vi "PicoScope6000aExampleRapidBlockBulk.vi"() -> ()   [LabVIEW 2016]
uses:
  <vilib>/Waveform/DWDTOps.llb/DWDT Analog to Digital.vi
  PicoScope6000aLib/PicoScope6000aAnalogChannelSettings.ctl
  PicoScope6000aLib/PicoScope6000aDigitalChannelSettings.ctl
panel:
  in  "Digital Channels":T1={"Port 0 Settings "={"Enabled"=FALSE, "Hysteresis"=3, "Threshold Level (Volts)"=[1.0, 1.0, 1.0, 1.0, 1.0, 1.0, 1.0, 1.0]}, "Port 1 Settings"={"Enabled"=FALSE, "Hysteresis"=3, "Threshold Level (Volts)"=[1.0, 1.0, 1.0, 1.0, 1.0, 1.0, 1.0, 1.0]}} {"Port 1 Settings"."Threshold Level (Volts)" format="%#_4p"; "Port 1 Settings"."Hysteresis" items=["PICO_VERY_HIGH_400MV", "PICO_HIGH_200MV", "PICO_NORMAL_100MV", "PICO_LOW_50MV"]; "Port 0 Settings"."Threshold Level (Volts)" format="%#_4p"; "Port 0 Settings"."Hysteresis" items=["PICO_VERY_HIGH_400MV", "PICO_HIGH_200MV", "PICO_NORMAL_100MV", "PICO_LOW_50MV"]}
  in  "Channels":T2={"Channel A Settings "={"Enabled"=FALSE, "Coupling"=1, "Range"=0, "Analogue Offset"=0.0, "BandWidth"=0}, "Channel B Settings "={"Enabled"=FALSE, "Coupling"=1, "Range"=0, "Analogue Offset"=0.0, "BandWidth"=0}, "Channel C Settings "={"Enabled"=FALSE, "Coupling"=1, "Range"=0, "Analogue Offset"=0.0, "BandWidth"=0}, "Channel D Settings "={"Enabled"=FALSE, "Coupling"=1, "Range"=0, "Analogue Offset"=0.0, "BandWidth"=0}, "Channel E Settings "={"Enabled"=FALSE, "Coupling"=1, "Range"=0, "Analogue Offset"=0.0, "BandWidth"=0}, "Channel F Settings "={"Enabled"=FALSE, "Coupling"=1, "Range"=0, "Analogue Offset"=0.0, "BandWidth"=0}, "Channel G Settings "={"Enabled"=FALSE, "Coupling"=1, "Range"=0, "Analogue Offset"=0.0, "BandWidth"=0}, "Channel H Settings "={"Enabled"=FALSE, "Coupling"=1, "Range"=0, "Analogue Offset"=0.0, "BandWidth"=0}} {"Channel H Settings"."BandWidth" items=["Full"=0, "100kHz"=100000, "20kHz"=200000, "1MHz"=1000000, "20MHz"=20000000, "25MHz"=25000000, "50MHz"=50000000, "200MHz"=200000000, "250MHz"=250000000, "500MHz"=500000000]; "Channel H Settings"."Range" items=["10mV"=0, "20mV"=1, "50mV"=2, "100mV"=3, "200mV"=4, "500mV"=5, "1V"=6, "2V"=7, "5V"=8, "10V"=9, "20V"=10, "50V"=11, "100V"=12, "200V"=13, "x10_Probe_100mV"=32, "x10_Probe_200mV"=33, "x10_Probe_500mV"=34, "x10_Probe_1V"=35, "x10_Probe_2V"=36, "x10_Probe_5V"=37, "x10_Probe_10V"=38, "x10_Probe_20V"=39, "x10_Probe_50V"=40, "x10_Probe_100V"=41, "x10_Probe_200V"=42, "x10_Probe_500V"=43, "CURRENT_CLAMP_60A_2A"=10500, "CURRENT_CLAMP_60A_5A"=10501, "CURRENT_CLAMP_60A_10A"=10502, "CURRENT_CLAMP_60A_20A"=10503, "CURRENT_CLAMP_60A_50A"=10504, "CURRENT_CLAMP_60A_60A"=10505, "CURRENT_CLAMP_60A_V2_0_5A"=10600, "CURRENT_CLAMP_60A_V2_1A"=10601, "CURRENT_CLAMP_60A_V2_2A"=10602, "CURRENT_CLAMP_60A_V2_5A"=10603, "CURRENT_CLAMP_60A_V2_10A"=10604, "CURRENT_CLAMP_60A_V2_20A"=10605, "CURRENT_CLAMP_60A_V2_50A"=10606, "CURRENT_CLAMP_60A_V2_60A"=10607, "RESISTANCE_LEAD_NEG5_TO_20OHM"=7000, "RESISTANCE_LEAD_NEG50_TO_200OHM"=7001, "RESISTANCE_LEAD_NEG500_TO_2KOHM"=7002, "RESISTANCE_LEAD_NEG5K_TO_20KOHM"=7003, "RESISTANCE_LEAD_NEG50K_TO_LEAD_200KOHM"=7004, "RESISTANCE_LEAD_NEG500K_TO_LEAD_2MOHM"=7005, "RESISTANCE_LEAD_DIODE_TEST"=7006, "HT_NEG3_TO_5KV"=8950, "HT_NEG3_TO_10KV"=8951, "HT_NEG5_TO_20KV"=8952, "HT_NEG5_TO_50KV"=8953, "HT_NEG5_TO_100KV"=8954, "HT_NEG3_TO_5KV_INVERTED"=8955, "HT_NEG3_TO_10KV_INVERTED"=8956, "HT_NEG5_TO_20KV_INVERTED"=8957, "HT_NEG5_TO_50KV_INVERTED"=8958, "HT_NEG5_TO_100KV_INVERTED"=8959, "TEMPERATURE_NEG50_TO_150DEGC"=9000, "PRESSURE_SENSOR_-100k-150k_PASCALS"=9100, "PRESSURE_SENSOR_-100k_TO_400k_PASCALS"=9101, "PRESSURE_SENSOR_-200k_TO_800k_PASCALS"=9102, "PRESSURE_SENSOR_-400k_TO_1600k_PASCALS"=9103, "PRESSURE_SENSOR_-400k_TO_3400k_PASCALS"=9104, "PRESSURE_SENSOR_-150k_TO_1350k_PASCALS"=9105]; "Channel H Settings"."Coupling" items=["AC"=0, "DC 1M Ohm"=1, "DC 50 Ohm"=50]; "Channel G Settings"."BandWidth" items=["Full"=0, "100kHz"=100000, "20kHz"=200000, "1MHz"=1000000, "20MHz"=20000000, "25MHz"=25000000, "50MHz"=50000000, "200MHz"=200000000, "250MHz"=250000000, "500MHz"=500000000]; "Channel G Settings"."Range" items=["10mV"=0, "20mV"=1, "50mV"=2, "100mV"=3, "200mV"=4, "500mV"=5, "1V"=6, "2V"=7, "5V"=8, "10V"=9, "20V"=10, "50V"=11, "100V"=12, "200V"=13, "x10_Probe_100mV"=32, "x10_Probe_200mV"=33, "x10_Probe_500mV"=34, "x10_Probe_1V"=35, "x10_Probe_2V"=36, "x10_Probe_5V"=37, "x10_Probe_10V"=38, "x10_Probe_20V"=39, "x10_Probe_50V"=40, "x10_Probe_100V"=41, "x10_Probe_200V"=42, "x10_Probe_500V"=43, "CURRENT_CLAMP_60A_2A"=10500, "CURRENT_CLAMP_60A_5A"=10501, "CURRENT_CLAMP_60A_10A"=10502, "CURRENT_CLAMP_60A_20A"=10503, "CURRENT_CLAMP_60A_50A"=10504, "CURRENT_CLAMP_60A_60A"=10505, "CURRENT_CLAMP_60A_V2_0_5A"=10600, "CURRENT_CLAMP_60A_V2_1A"=10601, "CURRENT_CLAMP_60A_V2_2A"=10602, "CURRENT_CLAMP_60A_V2_5A"=10603, "CURRENT_CLAMP_60A_V2_10A"=10604, "CURRENT_CLAMP_60A_V2_20A"=10605, "CURRENT_CLAMP_60A_V2_50A"=10606, "CURRENT_CLAMP_60A_V2_60A"=10607, "RESISTANCE_LEAD_NEG5_TO_20OHM"=7000, "RESISTANCE_LEAD_NEG50_TO_200OHM"=7001, "RESISTANCE_LEAD_NEG500_TO_2KOHM"=7002, "RESISTANCE_LEAD_NEG5K_TO_20KOHM"=7003, "RESISTANCE_LEAD_NEG50K_TO_LEAD_200KOHM"=7004, "RESISTANCE_LEAD_NEG500K_TO_LEAD_2MOHM"=7005, "RESISTANCE_LEAD_DIODE_TEST"=7006, "HT_NEG3_TO_5KV"=8950, "HT_NEG3_TO_10KV"=8951, "HT_NEG5_TO_20KV"=8952, "HT_NEG5_TO_50KV"=8953, "HT_NEG5_TO_100KV"=8954, "HT_NEG3_TO_5KV_INVERTED"=8955, "HT_NEG3_TO_10KV_INVERTED"=8956, "HT_NEG5_TO_20KV_INVERTED"=8957, "HT_NEG5_TO_50KV_INVERTED"=8958, "HT_NEG5_TO_100KV_INVERTED"=8959, "TEMPERATURE_NEG50_TO_150DEGC"=9000, "PRESSURE_SENSOR_-100k-150k_PASCALS"=9100, "PRESSURE_SENSOR_-100k_TO_400k_PASCALS"=9101, "PRESSURE_SENSOR_-200k_TO_800k_PASCALS"=9102, "PRESSURE_SENSOR_-400k_TO_1600k_PASCALS"=9103, "PRESSURE_SENSOR_-400k_TO_3400k_PASCALS"=9104, "PRESSURE_SENSOR_-150k_TO_1350k_PASCALS"=9105]; "Channel G Settings"."Coupling" items=["AC"=0, "DC 1M Ohm"=1, "DC 50 Ohm"=50]; "Channel F Settings"."BandWidth" items=["Full"=0, "100kHz"=100000, "20kHz"=200000, "1MHz"=1000000, "20MHz"=20000000, "25MHz"=25000000, "50MHz"=50000000, "200MHz"=200000000, "250MHz"=250000000, "500MHz"=500000000]; "Channel F Settings"."Range" items=["10mV"=0, "20mV"=1, "50mV"=2, "100mV"=3, "200mV"=4, "500mV"=5, "1V"=6, "2V"=7, "5V"=8, "10V"=9, "20V"=10, "50V"=11, "100V"=12, "200V"=13, "x10_Probe_100mV"=32, "x10_Probe_200mV"=33, "x10_Probe_500mV"=34, "x10_Probe_1V"=35, "x10_Probe_2V"=36, "x10_Probe_5V"=37, "x10_Probe_10V"=38, "x10_Probe_20V"=39, "x10_Probe_50V"=40, "x10_Probe_100V"=41, "x10_Probe_200V"=42, "x10_Probe_500V"=43, "CURRENT_CLAMP_60A_2A"=10500, "CURRENT_CLAMP_60A_5A"=10501, "CURRENT_CLAMP_60A_10A"=10502, "CURRENT_CLAMP_60A_20A"=10503, "CURRENT_CLAMP_60A_50A"=10504, "CURRENT_CLAMP_60A_60A"=10505, "CURRENT_CLAMP_60A_V2_0_5A"=10600, "CURRENT_CLAMP_60A_V2_1A"=10601, "CURRENT_CLAMP_60A_V2_2A"=10602, "CURRENT_CLAMP_60A_V2_5A"=10603, "CURRENT_CLAMP_60A_V2_10A"=10604, "CURRENT_CLAMP_60A_V2_20A"=10605, "CURRENT_CLAMP_60A_V2_50A"=10606, "CURRENT_CLAMP_60A_V2_60A"=10607, "RESISTANCE_LEAD_NEG5_TO_20OHM"=7000, "RESISTANCE_LEAD_NEG50_TO_200OHM"=7001, "RESISTANCE_LEAD_NEG500_TO_2KOHM"=7002, "RESISTANCE_LEAD_NEG5K_TO_20KOHM"=7003, "RESISTANCE_LEAD_NEG50K_TO_LEAD_200KOHM"=7004, "RESISTANCE_LEAD_NEG500K_TO_LEAD_2MOHM"=7005, "RESISTANCE_LEAD_DIODE_TEST"=7006, "HT_NEG3_TO_5KV"=8950, "HT_NEG3_TO_10KV"=8951, "HT_NEG5_TO_20KV"=8952, "HT_NEG5_TO_50KV"=8953, "HT_NEG5_TO_100KV"=8954, "HT_NEG3_TO_5KV_INVERTED"=8955, "HT_NEG3_TO_10KV_INVERTED"=8956, "HT_NEG5_TO_20KV_INVERTED"=8957, "HT_NEG5_TO_50KV_INVERTED"=8958, "HT_NEG5_TO_100KV_INVERTED"=8959, "TEMPERATURE_NEG50_TO_150DEGC"=9000, "PRESSURE_SENSOR_-100k-150k_PASCALS"=9100, "PRESSURE_SENSOR_-100k_TO_400k_PASCALS"=9101, "PRESSURE_SENSOR_-200k_TO_800k_PASCALS"=9102, "PRESSURE_SENSOR_-400k_TO_1600k_PASCALS"=9103, "PRESSURE_SENSOR_-400k_TO_3400k_PASCALS"=9104, "PRESSURE_SENSOR_-150k_TO_1350k_PASCALS"=9105]; "Channel F Settings"."Coupling" items=["AC"=0, "DC 1M Ohm"=1, "DC 50 Ohm"=50]; "Channel E Settings"."BandWidth" items=["Full"=0, "100kHz"=100000, "20kHz"=200000, "1MHz"=1000000, "20MHz"=20000000, "25MHz"=25000000, "50MHz"=50000000, "200MHz"=200000000, "250MHz"=250000000, "500MHz"=500000000]; "Channel E Settings"."Range" items=["10mV"=0, "20mV"=1, "50mV"=2, "100mV"=3, "200mV"=4, "500mV"=5, "1V"=6, "2V"=7, "5V"=8, "10V"=9, "20V"=10, "50V"=11, "100V"=12, "200V"=13, "x10_Probe_100mV"=32, "x10_Probe_200mV"=33, "x10_Probe_500mV"=34, "x10_Probe_1V"=35, "x10_Probe_2V"=36, "x10_Probe_5V"=37, "x10_Probe_10V"=38, "x10_Probe_20V"=39, "x10_Probe_50V"=40, "x10_Probe_100V"=41, "x10_Probe_200V"=42, "x10_Probe_500V"=43, "CURRENT_CLAMP_60A_2A"=10500, "CURRENT_CLAMP_60A_5A"=10501, "CURRENT_CLAMP_60A_10A"=10502, "CURRENT_CLAMP_60A_20A"=10503, "CURRENT_CLAMP_60A_50A"=10504, "CURRENT_CLAMP_60A_60A"=10505, "CURRENT_CLAMP_60A_V2_0_5A"=10600, "CURRENT_CLAMP_60A_V2_1A"=10601, "CURRENT_CLAMP_60A_V2_2A"=10602, "CURRENT_CLAMP_60A_V2_5A"=10603, "CURRENT_CLAMP_60A_V2_10A"=10604, "CURRENT_CLAMP_60A_V2_20A"=10605, "CURRENT_CLAMP_60A_V2_50A"=10606, "CURRENT_CLAMP_60A_V2_60A"=10607, "RESISTANCE_LEAD_NEG5_TO_20OHM"=7000, "RESISTANCE_LEAD_NEG50_TO_200OHM"=7001, "RESISTANCE_LEAD_NEG500_TO_2KOHM"=7002, "RESISTANCE_LEAD_NEG5K_TO_20KOHM"=7003, "RESISTANCE_LEAD_NEG50K_TO_LEAD_200KOHM"=7004, "RESISTANCE_LEAD_NEG500K_TO_LEAD_2MOHM"=7005, "RESISTANCE_LEAD_DIODE_TEST"=7006, "HT_NEG3_TO_5KV"=8950, "HT_NEG3_TO_10KV"=8951, "HT_NEG5_TO_20KV"=8952, "HT_NEG5_TO_50KV"=8953, "HT_NEG5_TO_100KV"=8954, "HT_NEG3_TO_5KV_INVERTED"=8955, "HT_NEG3_TO_10KV_INVERTED"=8956, "HT_NEG5_TO_20KV_INVERTED"=8957, "HT_NEG5_TO_50KV_INVERTED"=8958, "HT_NEG5_TO_100KV_INVERTED"=8959, "TEMPERATURE_NEG50_TO_150DEGC"=9000, "PRESSURE_SENSOR_-100k-150k_PASCALS"=9100, "PRESSURE_SENSOR_-100k_TO_400k_PASCALS"=9101, "PRESSURE_SENSOR_-200k_TO_800k_PASCALS"=9102, "PRESSURE_SENSOR_-400k_TO_1600k_PASCALS"=9103, "PRESSURE_SENSOR_-400k_TO_3400k_PASCALS"=9104, "PRESSURE_SENSOR_-150k_TO_1350k_PASCALS"=9105]; "Channel E Settings"."Coupling" items=["AC"=0, "DC 1M Ohm"=1, "DC 50 Ohm"=50]; "Channel D Settings"."BandWidth" items=["Full"=0, "100kHz"=100000, "20kHz"=200000, "1MHz"=1000000, "20MHz"=20000000, "25MHz"=25000000, "50MHz"=50000000, "200MHz"=200000000, "250MHz"=250000000, "500MHz"=500000000]; "Channel D Settings"."Range" items=["10mV"=0, "20mV"=1, "50mV"=2, "100mV"=3, "200mV"=4, "500mV"=5, "1V"=6, "2V"=7, "5V"=8, "10V"=9, "20V"=10, "50V"=11, "100V"=12, "200V"=13, "x10_Probe_100mV"=32, "x10_Probe_200mV"=33, "x10_Probe_500mV"=34, "x10_Probe_1V"=35, "x10_Probe_2V"=36, "x10_Probe_5V"=37, "x10_Probe_10V"=38, "x10_Probe_20V"=39, "x10_Probe_50V"=40, "x10_Probe_100V"=41, "x10_Probe_200V"=42, "x10_Probe_500V"=43, "CURRENT_CLAMP_60A_2A"=10500, "CURRENT_CLAMP_60A_5A"=10501, "CURRENT_CLAMP_60A_10A"=10502, "CURRENT_CLAMP_60A_20A"=10503, "CURRENT_CLAMP_60A_50A"=10504, "CURRENT_CLAMP_60A_60A"=10505, "CURRENT_CLAMP_60A_V2_0_5A"=10600, "CURRENT_CLAMP_60A_V2_1A"=10601, "CURRENT_CLAMP_60A_V2_2A"=10602, "CURRENT_CLAMP_60A_V2_5A"=10603, "CURRENT_CLAMP_60A_V2_10A"=10604, "CURRENT_CLAMP_60A_V2_20A"=10605, "CURRENT_CLAMP_60A_V2_50A"=10606, "CURRENT_CLAMP_60A_V2_60A"=10607, "RESISTANCE_LEAD_NEG5_TO_20OHM"=7000, "RESISTANCE_LEAD_NEG50_TO_200OHM"=7001, "RESISTANCE_LEAD_NEG500_TO_2KOHM"=7002, "RESISTANCE_LEAD_NEG5K_TO_20KOHM"=7003, "RESISTANCE_LEAD_NEG50K_TO_LEAD_200KOHM"=7004, "RESISTANCE_LEAD_NEG500K_TO_LEAD_2MOHM"=7005, "RESISTANCE_LEAD_DIODE_TEST"=7006, "HT_NEG3_TO_5KV"=8950, "HT_NEG3_TO_10KV"=8951, "HT_NEG5_TO_20KV"=8952, "HT_NEG5_TO_50KV"=8953, "HT_NEG5_TO_100KV"=8954, "HT_NEG3_TO_5KV_INVERTED"=8955, "HT_NEG3_TO_10KV_INVERTED"=8956, "HT_NEG5_TO_20KV_INVERTED"=8957, "HT_NEG5_TO_50KV_INVERTED"=8958, "HT_NEG5_TO_100KV_INVERTED"=8959, "TEMPERATURE_NEG50_TO_150DEGC"=9000, "PRESSURE_SENSOR_-100k-150k_PASCALS"=9100, "PRESSURE_SENSOR_-100k_TO_400k_PASCALS"=9101, "PRESSURE_SENSOR_-200k_TO_800k_PASCALS"=9102, "PRESSURE_SENSOR_-400k_TO_1600k_PASCALS"=9103, "PRESSURE_SENSOR_-400k_TO_3400k_PASCALS"=9104, "PRESSURE_SENSOR_-150k_TO_1350k_PASCALS"=9105]; "Channel D Settings"."Coupling" items=["AC"=0, "DC 1M Ohm"=1, "DC 50 Ohm"=50]; "Channel C Settings"."BandWidth" items=["Full"=0, "100kHz"=100000, "20kHz"=200000, "1MHz"=1000000, "20MHz"=20000000, "25MHz"=25000000, "50MHz"=50000000, "200MHz"=200000000, "250MHz"=250000000, "500MHz"=500000000]; "Channel C Settings"."Range" items=["10mV"=0, "20mV"=1, "50mV"=2, "100mV"=3, "200mV"=4, "500mV"=5, "1V"=6, "2V"=7, "5V"=8, "10V"=9, "20V"=10, "50V"=11, "100V"=12, "200V"=13, "x10_Probe_100mV"=32, "x10_Probe_200mV"=33, "x10_Probe_500mV"=34, "x10_Probe_1V"=35, "x10_Probe_2V"=36, "x10_Probe_5V"=37, "x10_Probe_10V"=38, "x10_Probe_20V"=39, "x10_Probe_50V"=40, "x10_Probe_100V"=41, "x10_Probe_200V"=42, "x10_Probe_500V"=43, "CURRENT_CLAMP_60A_2A"=10500, "CURRENT_CLAMP_60A_5A"=10501, "CURRENT_CLAMP_60A_10A"=10502, "CURRENT_CLAMP_60A_20A"=10503, "CURRENT_CLAMP_60A_50A"=10504, "CURRENT_CLAMP_60A_60A"=10505, "CURRENT_CLAMP_60A_V2_0_5A"=10600, "CURRENT_CLAMP_60A_V2_1A"=10601, "CURRENT_CLAMP_60A_V2_2A"=10602, "CURRENT_CLAMP_60A_V2_5A"=10603, "CURRENT_CLAMP_60A_V2_10A"=10604, "CURRENT_CLAMP_60A_V2_20A"=10605, "CURRENT_CLAMP_60A_V2_50A"=10606, "CURRENT_CLAMP_60A_V2_60A"=10607, "RESISTANCE_LEAD_NEG5_TO_20OHM"=7000, "RESISTANCE_LEAD_NEG50_TO_200OHM"=7001, "RESISTANCE_LEAD_NEG500_TO_2KOHM"=7002, "RESISTANCE_LEAD_NEG5K_TO_20KOHM"=7003, "RESISTANCE_LEAD_NEG50K_TO_LEAD_200KOHM"=7004, "RESISTANCE_LEAD_NEG500K_TO_LEAD_2MOHM"=7005, "RESISTANCE_LEAD_DIODE_TEST"=7006, "HT_NEG3_TO_5KV"=8950, "HT_NEG3_TO_10KV"=8951, "HT_NEG5_TO_20KV"=8952, "HT_NEG5_TO_50KV"=8953, "HT_NEG5_TO_100KV"=8954, "HT_NEG3_TO_5KV_INVERTED"=8955, "HT_NEG3_TO_10KV_INVERTED"=8956, "HT_NEG5_TO_20KV_INVERTED"=8957, "HT_NEG5_TO_50KV_INVERTED"=8958, "HT_NEG5_TO_100KV_INVERTED"=8959, "TEMPERATURE_NEG50_TO_150DEGC"=9000, "PRESSURE_SENSOR_-100k-150k_PASCALS"=9100, "PRESSURE_SENSOR_-100k_TO_400k_PASCALS"=9101, "PRESSURE_SENSOR_-200k_TO_800k_PASCALS"=9102, "PRESSURE_SENSOR_-400k_TO_1600k_PASCALS"=9103, "PRESSURE_SENSOR_-400k_TO_3400k_PASCALS"=9104, "PRESSURE_SENSOR_-150k_TO_1350k_PASCALS"=9105]; "Channel C Settings"."Coupling" items=["AC"=0, "DC 1M Ohm"=1, "DC 50 Ohm"=50]; "Channel B Settings"."BandWidth" items=["Full"=0, "100kHz"=100000, "20kHz"=200000, "1MHz"=1000000, "20MHz"=20000000, "25MHz"=25000000, "50MHz"=50000000, "200MHz"=200000000, "250MHz"=250000000, "500MHz"=500000000]; "Channel B Settings"."Range" items=["10mV"=0, "20mV"=1, "50mV"=2, "100mV"=3, "200mV"=4, "500mV"=5, "1V"=6, "2V"=7, "5V"=8, "10V"=9, "20V"=10, "50V"=11, "100V"=12, "200V"=13, "x10_Probe_100mV"=32, "x10_Probe_200mV"=33, "x10_Probe_500mV"=34, "x10_Probe_1V"=35, "x10_Probe_2V"=36, "x10_Probe_5V"=37, "x10_Probe_10V"=38, "x10_Probe_20V"=39, "x10_Probe_50V"=40, "x10_Probe_100V"=41, "x10_Probe_200V"=42, "x10_Probe_500V"=43, "CURRENT_CLAMP_60A_2A"=10500, "CURRENT_CLAMP_60A_5A"=10501, "CURRENT_CLAMP_60A_10A"=10502, "CURRENT_CLAMP_60A_20A"=10503, "CURRENT_CLAMP_60A_50A"=10504, "CURRENT_CLAMP_60A_60A"=10505, "CURRENT_CLAMP_60A_V2_0_5A"=10600, "CURRENT_CLAMP_60A_V2_1A"=10601, "CURRENT_CLAMP_60A_V2_2A"=10602, "CURRENT_CLAMP_60A_V2_5A"=10603, "CURRENT_CLAMP_60A_V2_10A"=10604, "CURRENT_CLAMP_60A_V2_20A"=10605, "CURRENT_CLAMP_60A_V2_50A"=10606, "CURRENT_CLAMP_60A_V2_60A"=10607, "RESISTANCE_LEAD_NEG5_TO_20OHM"=7000, "RESISTANCE_LEAD_NEG50_TO_200OHM"=7001, "RESISTANCE_LEAD_NEG500_TO_2KOHM"=7002, "RESISTANCE_LEAD_NEG5K_TO_20KOHM"=7003, "RESISTANCE_LEAD_NEG50K_TO_LEAD_200KOHM"=7004, "RESISTANCE_LEAD_NEG500K_TO_LEAD_2MOHM"=7005, "RESISTANCE_LEAD_DIODE_TEST"=7006, "HT_NEG3_TO_5KV"=8950, "HT_NEG3_TO_10KV"=8951, "HT_NEG5_TO_20KV"=8952, "HT_NEG5_TO_50KV"=8953, "HT_NEG5_TO_100KV"=8954, "HT_NEG3_TO_5KV_INVERTED"=8955, "HT_NEG3_TO_10KV_INVERTED"=8956, "HT_NEG5_TO_20KV_INVERTED"=8957, "HT_NEG5_TO_50KV_INVERTED"=8958, "HT_NEG5_TO_100KV_INVERTED"=8959, "TEMPERATURE_NEG50_TO_150DEGC"=9000, "PRESSURE_SENSOR_-100k-150k_PASCALS"=9100, "PRESSURE_SENSOR_-100k_TO_400k_PASCALS"=9101, "PRESSURE_SENSOR_-200k_TO_800k_PASCALS"=9102, "PRESSURE_SENSOR_-400k_TO_1600k_PASCALS"=9103, "PRESSURE_SENSOR_-400k_TO_3400k_PASCALS"=9104, "PRESSURE_SENSOR_-150k_TO_1350k_PASCALS"=9105]; "Channel B Settings"."Coupling" items=["AC"=0, "DC 1M Ohm"=1, "DC 50 Ohm"=50]; "Channel A Settings"."Range" items=["10mV"=0, "20mV"=1, "50mV"=2, "100mV"=3, "200mV"=4, "500mV"=5, "1V"=6, "2V"=7, "5V"=8, "10V"=9, "20V"=10, "50V"=11, "100V"=12, "200V"=13, "x10_Probe_100mV"=32, "x10_Probe_200mV"=33, "x10_Probe_500mV"=34, "x10_Probe_1V"=35, "x10_Probe_2V"=36, "x10_Probe_5V"=37, "x10_Probe_10V"=38, "x10_Probe_20V"=39, "x10_Probe_50V"=40, "x10_Probe_100V"=41, "x10_Probe_200V"=42, "x10_Probe_500V"=43, "CURRENT_CLAMP_60A_2A"=10500, "CURRENT_CLAMP_60A_5A"=10501, "CURRENT_CLAMP_60A_10A"=10502, "CURRENT_CLAMP_60A_20A"=10503, "CURRENT_CLAMP_60A_50A"=10504, "CURRENT_CLAMP_60A_60A"=10505, "CURRENT_CLAMP_60A_V2_0_5A"=10600, "CURRENT_CLAMP_60A_V2_1A"=10601, "CURRENT_CLAMP_60A_V2_2A"=10602, "CURRENT_CLAMP_60A_V2_5A"=10603, "CURRENT_CLAMP_60A_V2_10A"=10604, "CURRENT_CLAMP_60A_V2_20A"=10605, "CURRENT_CLAMP_60A_V2_50A"=10606, "CURRENT_CLAMP_60A_V2_60A"=10607, "RESISTANCE_LEAD_NEG5_TO_20OHM"=7000, "RESISTANCE_LEAD_NEG50_TO_200OHM"=7001, "RESISTANCE_LEAD_NEG500_TO_2KOHM"=7002, "RESISTANCE_LEAD_NEG5K_TO_20KOHM"=7003, "RESISTANCE_LEAD_NEG50K_TO_LEAD_200KOHM"=7004, "RESISTANCE_LEAD_NEG500K_TO_LEAD_2MOHM"=7005, "RESISTANCE_LEAD_DIODE_TEST"=7006, "HT_NEG3_TO_5KV"=8950, "HT_NEG3_TO_10KV"=8951, "HT_NEG5_TO_20KV"=8952, "HT_NEG5_TO_50KV"=8953, "HT_NEG5_TO_100KV"=8954, "HT_NEG3_TO_5KV_INVERTED"=8955, "HT_NEG3_TO_10KV_INVERTED"=8956, "HT_NEG5_TO_20KV_INVERTED"=8957, "HT_NEG5_TO_50KV_INVERTED"=8958, "HT_NEG5_TO_100KV_INVERTED"=8959, "TEMPERATURE_NEG50_TO_150DEGC"=9000, "PRESSURE_SENSOR_-100k-150k_PASCALS"=9100, "PRESSURE_SENSOR_-100k_TO_400k_PASCALS"=9101, "PRESSURE_SENSOR_-200k_TO_800k_PASCALS"=9102, "PRESSURE_SENSOR_-400k_TO_1600k_PASCALS"=9103, "PRESSURE_SENSOR_-400k_TO_3400k_PASCALS"=9104, "PRESSURE_SENSOR_-150k_TO_1350k_PASCALS"=9105]; "Channel A Settings"."BandWidth" items=["Full"=0, "100kHz"=100000, "20kHz"=200000, "1MHz"=1000000, "20MHz"=20000000, "25MHz"=25000000, "50MHz"=50000000, "200MHz"=200000000, "250MHz"=250000000, "500MHz"=500000000]; "Channel A Settings"."Coupling" items=["AC"=0, "DC 1M Ohm"=1, "DC 50 Ohm"=50]}
  out "overflow":i16[](array[numeric]) format="%08b"
  out "nMaxSamples":u64 format="%#_6p"
  in  "Buffer and Transfer Settings":T3={"fromSegmentIndex"=0, "toSegmentIndex"=20, "startIndex"=0, "noOfSamples"=10000000, "Down-Sample Mode"=2147483648, "Down Sample Ratio"=10} {"Down-Sample Mode" items=["None"=2147483648, "Aggregate"=1, "Decimate"=2, "Average"=4]; "Down Sample Ratio" step=1; "noOfSamples" format="%#_6p"}
  in  "Acquisition Settings":T4={"preTriggerSamples"=0, "postTriggerSamples"=10000000, "timebase"=2, "Number of Captures"=20} {"postTriggerSamples" format="%#_6p"; "preTriggerSamples" format="%#_6p"}
  out "Capture Complete":bool
  out "Number of Samples \nPer Capture":u64 format="%#_6p"
  in  "Run":bool
  in  "Capture Index":i16 min=0
  out "Properties Panel":T5 {"Max Total Capture Time Available (sec)" format="%.3p"; "Sample Frequency" format="%.6p"; "Sample Rate" format="%.3p"; "Max Samples Available" format="%_6p"; "Total Capture Time (sec)" format="%.3p"}
  out "Port 0":digitalwaveform(graph)={"t0"=timestamp(0 s since 1904-01-01), "dt"=8e-09, "Y"={"transitions"=[], "data"=[]}}
  in  "Trigger Settings":T6={"Trigger Enabled"=FALSE, "Trigger Threshold (Volts)"=0.0, "Trigger Direction"=2, "Trigger Delay (samples)"=0, "Auto Trigger Time (us)"=100000, "Trigger Source"=0} {"Trigger Source" items=["Channel A"=0, "Channel B"=1, "Channel C"=2, "Channel D"=3, "Channel E"=4, "Channel F"=5, "Channel G"=6, "Channel H"=7, "Port 0"=128, "Port 1"=129, "Trigger AUX"=1001]; "Trigger Direction" items=["Rising"=2, "Falling"=3]; "Trigger Threshold (Volts)" format="%#_6p"}
  in  "stop":bool
  out "Analog Channels":cluster{i32, dbl, "Data (Volts)":dbl[]}[](graph)
  out "Device Info":T7={"PICO_DRIVER_VERSION"="", "PICO_USB_VERSION"="", "PICO_HARDWARE_VERSION"="", "PICO_VARIANT_INFO"="", "PICO_BATCH_AND_SERIAL"="", "PICO_CAL_DATE"="", "PICO_KERNEL_VERSION"="", "PICO_DIGITAL_HARDWARE_VERSION"="", "PICO_ANALOGUE_HARDWARE_VERSION"="", "PICO_FIRMWARE_VERSION_1"="", "PICO_FIRMWARE_VERSION_2"="", "PICO_IPP_VERSION"="", "PICO_DRIVER_PATH"="", "PICO_FIRMWARE_VERSION_3"="", "PICO_FRONT_PANEL_FIRMWARE_VERSION"="", "Number of Channels"=0, "MSO"=TRUE}
  out "Pico 6000a Units":string
  in  "Resolution":u32(ring) items=["8-bit"=0, "12-bit"=1, "14-bit"=2, "15-bit"=3, "16-bit"=4, "10-bit"=10]
  in  "Serial Number":string
  in  "Use Serial Number":bool
  in  "error in (no error)":errorcluster
  # "Please Ensure you set the \"Range\"(Probe type) before running the VI"
  # "D8-D15"
  # "DO-D7"
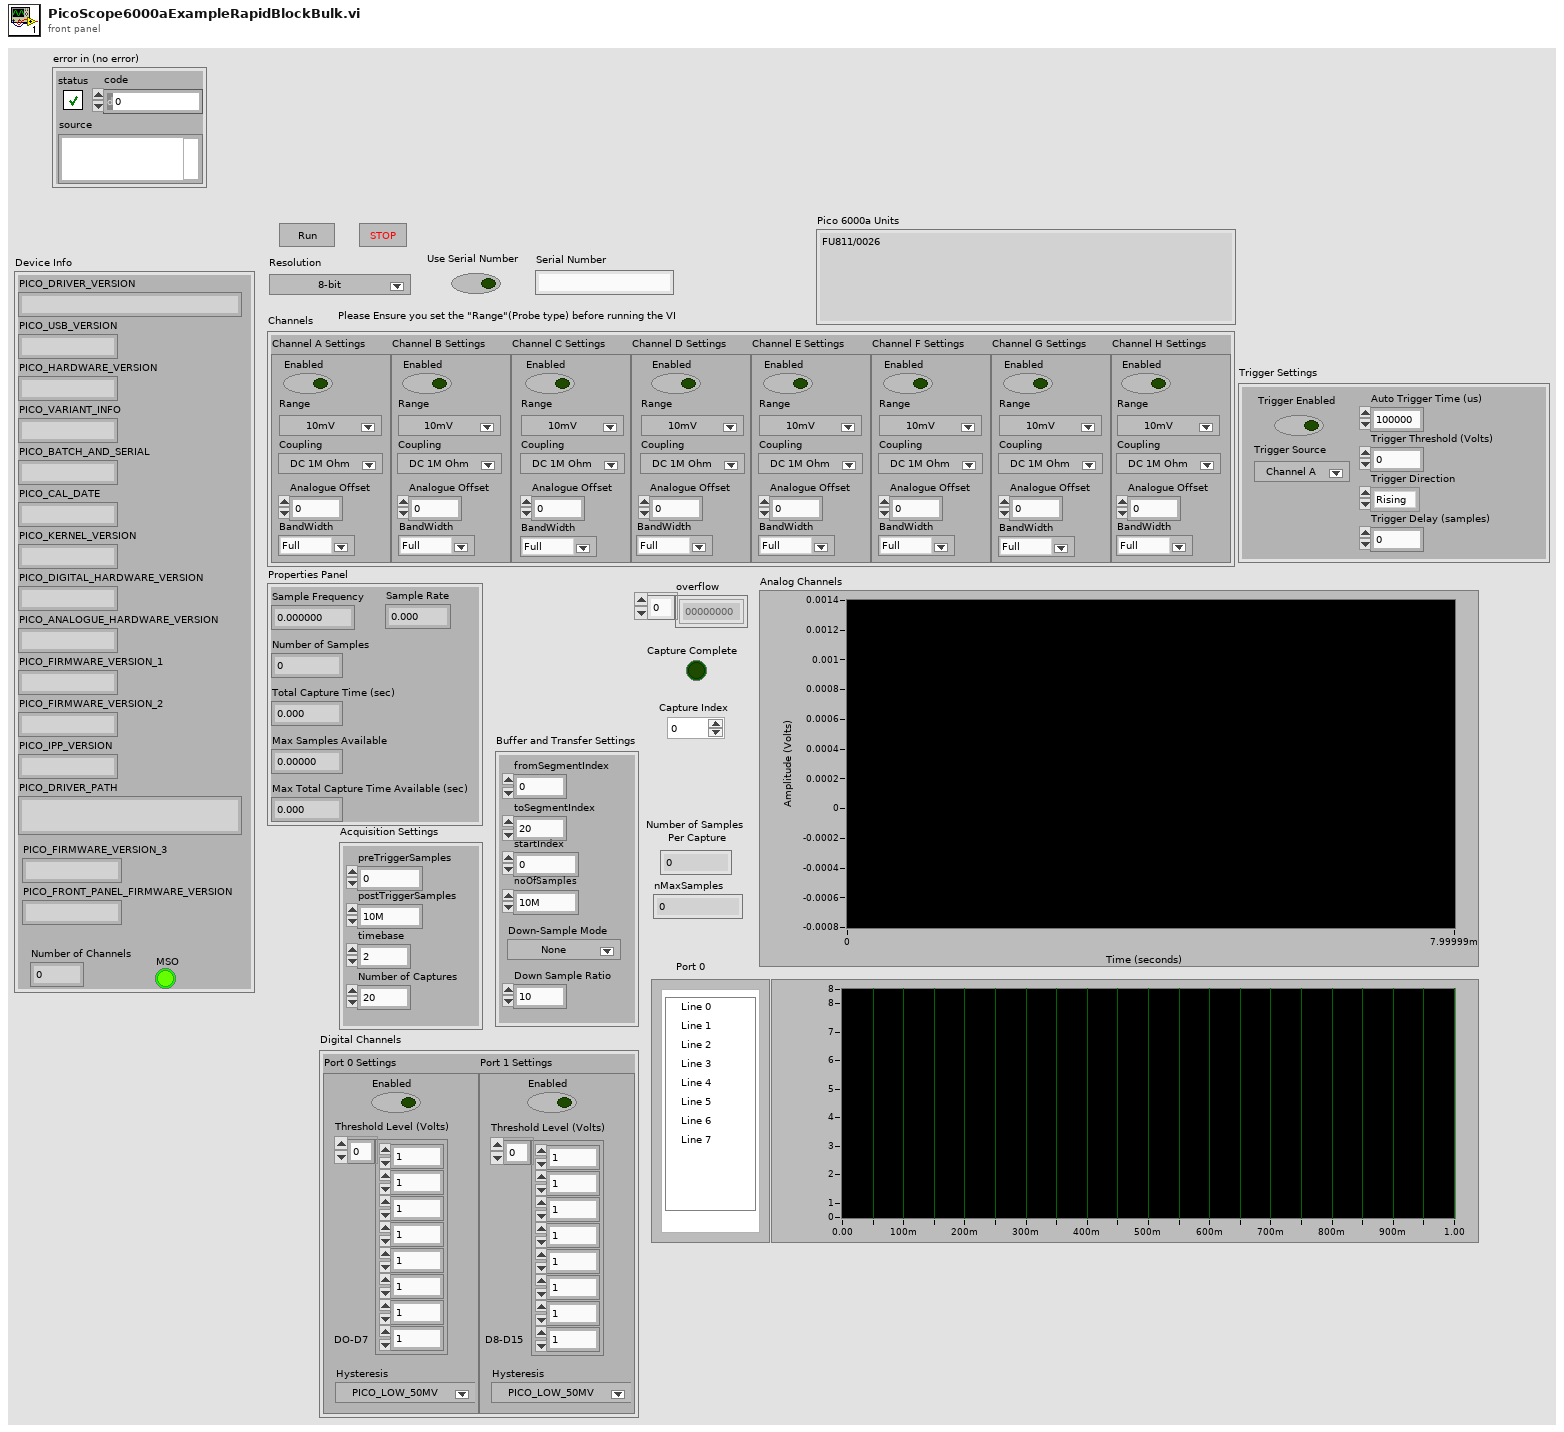
[diagram p1: front panel]
types:
  T1 = typedef "PicoScope6000aDigitalChannelSettings.ctl" = cluster{"Port 0 Settings ":cluster{"Enabled":bool, "Hysteresis":u32, "Threshold Level (Volts)":dbl[]}, "Port 1 Settings":cluster{"Enabled":bool, "Hysteresis":u32, "Threshold Level (Volts)":dbl[]}}
  T2 = typedef "PicoScope6000aAnalogChannelSettings.ctl" = cluster{"Channel A Settings ":cluster{"Enabled":bool, "Coupling":i16, "Range":u16, "Analogue Offset":dbl, "BandWidth":u32}, "Channel B Settings ":cluster{"Enabled":bool, "Coupling":i16, "Range":u16, "Analogue Offset":dbl, "BandWidth":u32}, "Channel C Settings ":cluster{"Enabled":bool, "Coupling":i16, "Range":u16, "Analogue Offset":dbl, "BandWidth":u32}, "Channel D Settings ":cluster{"Enabled":bool, "Coupling":i16, "Range":u16, "Analogue Offset":dbl, "BandWidth":u32}, "Channel E Settings ":cluster{"Enabled":bool, "Coupling":i16, "Range":u16, "Analogue Offset":dbl, "BandWidth":u32}, "Channel F Settings ":cluster{"Enabled":bool, "Coupling":i16, "Range":u16, "Analogue Offset":dbl, "BandWidth":u32}, "Channel G Settings ":cluster{"Enabled":bool, "Coupling":i16, "Range":u16, "Analogue Offset":dbl, "BandWidth":u32}, "Channel H Settings ":cluster{"Enabled":bool, "Coupling":i16, "Range":u16, "Analogue Offset":dbl, "BandWidth":u32}}
  T3 = cluster{"fromSegmentIndex":u64, "toSegmentIndex":u64, "startIndex":u64, "noOfSamples":u64, "Down-Sample Mode":u32, "Down Sample Ratio":u64}
  T4 = cluster{"preTriggerSamples":u64, "postTriggerSamples":u64, "timebase":u32, "Number of Captures":u64}
  T5 = cluster{"Sample Frequency":dbl, "Sample Rate":dbl, "Max Samples Available":u64, "Number of Samples":u64, "Total Capture Time (sec) ":dbl, "Max Total Capture Time Available (sec)":dbl}
  T6 = cluster{"Trigger Enabled":bool, "Trigger Threshold (Volts)":dbl, "Trigger Direction":u16, "Trigger Delay (samples)":u64, "Auto Trigger Time (us)":u32, "Trigger Source":u32}
  T7 = cluster{"PICO_DRIVER_VERSION":string, "PICO_USB_VERSION":string, "PICO_HARDWARE_VERSION":string, "PICO_VARIANT_INFO":string, "PICO_BATCH_AND_SERIAL":string, "PICO_CAL_DATE":string, "PICO_KERNEL_VERSION":string, "PICO_DIGITAL_HARDWARE_VERSION":string, "PICO_ANALOGUE_HARDWARE_VERSION":string, "PICO_FIRMWARE_VERSION_1":string, "PICO_FIRMWARE_VERSION_2":string, "PICO_IPP_VERSION":string, "PICO_DRIVER_PATH":string, "PICO_FIRMWARE_VERSION_3":string, "PICO_FRONT_PANEL_FIRMWARE_VERSION":string, "Number of Channels":i16, "MSO":bool}
  T8 = cluster{"bufferMax ChA":i16[][], "bufferMax ChB":i16[][], "bufferMax ChC":i16[][], "bufferMax ChD":i16[][], "bufferMax ChE":i16[][], "bufferMin ChF":i16[][], "bufferMin ChG":i16[][], "bufferMax ChH":i16[][], "bufferMax Port0":i16[][], "bufferMax Port1":i16[][]}
  T9 = cluster{"preTriggerSamples":u64, "postTriggerSamples":u64, "timebase":u32}
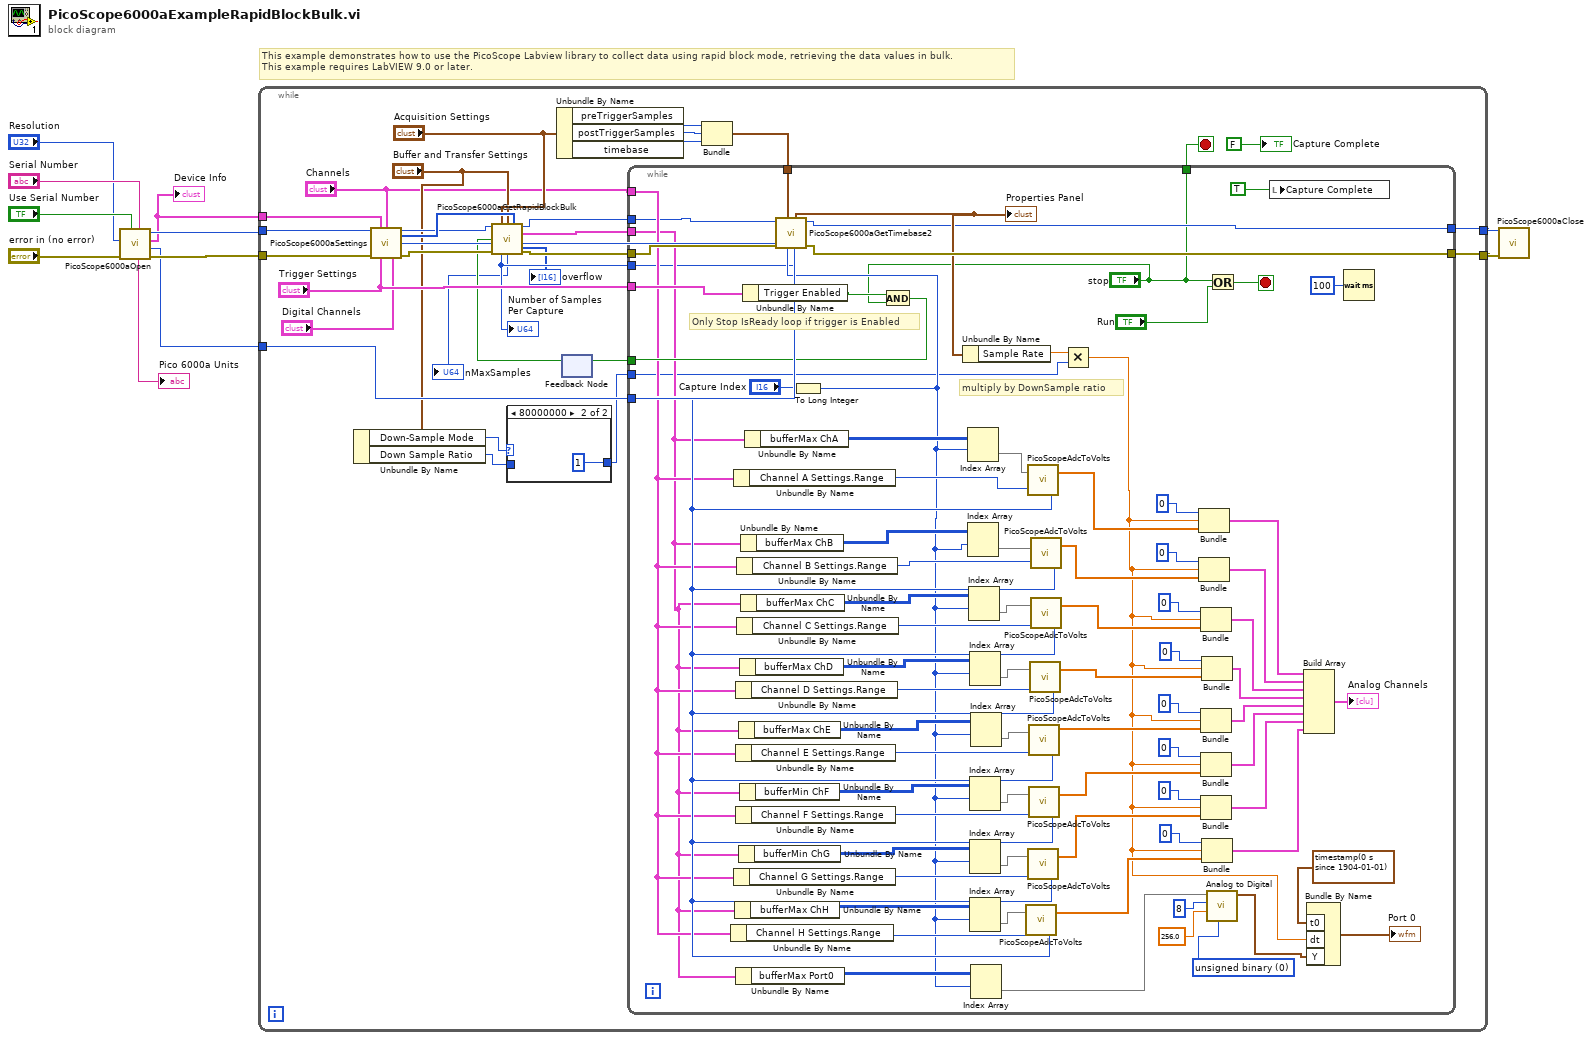
[diagram p0: block diagram]
diagram:
  # "This example demonstrates how to use the PicoScope Labview library to collect data using rapid block mode, retrieving the data values in bulk.\nThis example requires LabVIEW 9.0 or later."
  n1 = call "PicoScope6000aOpen.vi"("Serial Number"="Serial Number", "Use Serial Number"="Use Serial Number", "error in (no error)"="error in (no error)", "Resolution"="Resolution") -> ("error out"=w7:errorcluster, "Max ADC value"=w1:i16, "Device Info"=w2:T7, "handle out"=w8:i16, "Pico 6000a Units"=→"Pico 6000a Units":string)  [unwired: 2 in, 1 out]
  "Device Info" <- w2
  n2 = while {
    tunnel: w2 -> [w40]
    tunnel: w1 -> [w37]
    tunnel: w8 -> [w42]
    tunnel: [w35] -> w6
    tunnel: w7 -> [w41]
    tunnel: [w36] -> w5
    stop <- w31 stop-if-true
    n3 = Unbundle By Name("Buffer and Transfer Settings") -> ("Down-Sample Mode"=w18:u32, "Down Sample Ratio"=w17:u64)
    n4 = call "PicoScope6000aSettings.vi"("handle in"=w42, "Device Info"=w40, "Channels"="Channels", "Max ADC value"=w37, "error in (no error)"=w41, "Trigger Settings"="Trigger Settings", "Digital Channels"="Digital Channels") -> ("Enabled array"=w39:i16[], "handle out"=w28:i16, "error out"=w30:errorcluster)  [unwired: 6 in]
    n5 = case shown="80000000" w18 {
      tunnel: [w43 u64 1 ("Down Sample Ratio")] -> w16
      tunnel: w17 -> [w43 _]
      frame Default {
      }
      frame -2147483648 {
      }
    }
    n6 = Unbundle By Name("Acquisition Settings") -> ("preTriggerSamples"=w24:u64, "postTriggerSamples"=w23:u64, "timebase"=w22:u32)
    n7 = feedback #1() -> (w25:bool)  [unwired: 1 in]
    n8 = call "PicoScope6000aGetRapidBlockBulk.vi"("handle in"=w28, "Acquisition Settings"="Acquisition Settings", "Buffer and Transfer Settings"="Buffer and Transfer Settings", "enabled array"=w39, "stop IsReady"=w25, "error in (no error)"=w30) -> ("handle out"=w27:i16, "Buffers (Max or non-aggregated)"=w34:T8, "noOfSamples"=w33:u64, "nMaxSamples"=→"nMaxSamples":u64, "overflow"=→"overflow":i16[], "error out"=w29:errorcluster)  [unwired: 3 in, 1 out]
    "Number of Samples \nPer Capture" <- w33
    n9 = Bundle("preTriggerSamples"=w24, "postTriggerSamples"=w23, "timebase"=w22) -> (w21:T9)  [unwired: 1 in]
    n10 = while {
      tunnel: "Trigger Settings" -> [w85]
      tunnel: w37 -> [w83]
      tunnel: [w82] -> w26
      tunnel: "Channels" -> [w72]
      tunnel: w34 -> [w62]
      tunnel: w33 -> [w60]
      tunnel: [w75] -> w35
      tunnel: w27 -> [w57]
      tunnel: w29 -> [w78]
      tunnel: [w77] -> w36
      tunnel: ["stop"] -> w31
      tunnel: w21 -> [w54]
      tunnel: w16 -> [w45]
      stop <- w56 stop-if-true
      w90 = u16 0 items=["unsigned binary", "offset binary", "2's complement"] ("data format (offset binary)")
      # "multiply by DownSample ratio"
      # "Only Stop IsReady loop if trigger is Enabled"
      n11 = Unbundle By Name(w72) -> ("Channel H Settings.Range"=w110:u16)
      n12 = Unbundle By Name(w72) -> ("Channel A Settings.Range"=w123:u16)
      n13 = Unbundle By Name(w72) -> ("Channel G Settings.Range"=w111:u16)
      n14 = Unbundle By Name(w62) -> ("bufferMax ChH"=w69:i16[][])
      n15 = Unbundle By Name(w72) -> ("Channel D Settings.Range"=w114:u16)
      n16 = Unbundle By Name(w72) -> ("Channel E Settings.Range"=w113:u16)
      n17 = Unbundle By Name(w72) -> ("Channel F Settings.Range"=w112:u16)
      n18 = Unbundle By Name(w62) -> ("bufferMax Port0"=w73:i16[][])
      n19 = Unbundle By Name(w72) -> ("Channel B Settings.Range"=w121:u16)
      n20 = Unbundle By Name(w72) -> ("Channel C Settings.Range"=w115:u16)
      n21 = Unbundle By Name(w62) -> ("bufferMax ChE"=w66:i16[][])
      n22 = Unbundle By Name(w62) -> ("bufferMin ChG"=w68:i16[][])
      n23 = Unbundle By Name(w62) -> ("bufferMax ChD"=w65:i16[][])
      n24 = Unbundle By Name(w62) -> ("bufferMin ChF"=w67:i16[][])
      n25 = Unbundle By Name(w62) -> ("bufferMax ChB"=w70:i16[][])
      n26 = Unbundle By Name(w62) -> ("bufferMax ChC"=w64:i16[][])
      n27 = Unbundle By Name(w85) -> ("Trigger Enabled"=w84:bool)
      n28 = Unbundle By Name(w62) -> ("bufferMax ChA"=w80:i16[][])
      n29 = To Long Integer(number="Capture Index") -> (32bit integer=w63:i32)
      n30 = call "PicoScope6000aGetTimebase2.vi"("Number of Samples"=w60, "Memory Segment"=w63, "Acquisition Settings"=w54, "error in (no error)"=w78, "handle in"=w57) -> ("error out"=w77:errorcluster, "handle out"=w75:i16, "Properties Panel"=w76:T5)  [unwired: 4 in]
      "Properties Panel" <- w76
      n31 = And(x=w84, y="stop") -> (x .and. y?=w82:bool)
      n32 = Unbundle By Name(w76) -> ("Sample Rate"=w46:dbl)
      n33 = Index Array(array=w80, index (row)=w63) -> (element=w79:i16[])  [unwired: 1 in]
      n34 = Index Array(array=w70, index (row)=w63) -> (element=w71:i16[])  [unwired: 1 in]
      n35 = Index Array(array=w64, index (row)=w63) -> (element=w53:i16[])  [unwired: 1 in]
      n36 = Index Array(array=w65, index (row)=w63) -> (element=w52:i16[])  [unwired: 1 in]
      n37 = Index Array(array=w67, index (row)=w63) -> (element=w50:i16[])  [unwired: 1 in]
      n38 = Index Array(array=w68, index (row)=w63) -> (element=w49:i16[])  [unwired: 1 in]
      n39 = Index Array(array=w69, index (row)=w63) -> (element=w48:i16[])  [unwired: 1 in]
      n40 = Index Array(array=w66, index (row)=w63) -> (element=w51:i16[])  [unwired: 1 in]
      n41 = Index Array(array=w73, index (row)=w63) -> (element=w74:i16[])  [unwired: 1 in]
      n42 = call "PicoScopeAdcToVolts.vi"("Max_adc"=w83, "Range Index"=w110, "Data"=w48) -> ("Data"=w105:dbl[])
      n43 = call "PicoScopeAdcToVolts.vi"("Max_adc"=w83, "Range Index"=w123, "Data"=w79) -> ("Data"=w120:dbl[])
      n44 = call "PicoScopeAdcToVolts.vi"("Max_adc"=w83, "Range Index"=w111, "Data"=w49) -> ("Data"=w99:dbl[])
      n45 = call "PicoScopeAdcToVolts.vi"("Max_adc"=w83, "Range Index"=w113, "Data"=w51) -> ("Data"=w102:dbl[])
      n46 = call "PicoScopeAdcToVolts.vi"("Max_adc"=w83, "Range Index"=w112, "Data"=w50) -> ("Data"=w98:dbl[])
      n47 = call "PicoScopeAdcToVolts.vi"("Max_adc"=w83, "Range Index"=w114, "Data"=w52) -> ("Data"=w103:dbl[])
      n48 = call "PicoScopeAdcToVolts.vi"("Max_adc"=w83, "Range Index"=w121, "Data"=w71) -> ("Data"=w119:dbl[])
      n49 = call "PicoScopeAdcToVolts.vi"("Max_adc"=w83, "Range Index"=w115, "Data"=w53) -> ("Data"=w104:dbl[])
      n50 = Multiply(x=w46, y=w45) -> (x*y=w47:dbl)
      n51 = Bundle(0, w47, "Data"=w120) -> (w118:cluster{i32, dbl, "Data":dbl[]})  [unwired: 1 in]
      n52 = Bundle(0, w47, "Data"=w119) -> (w117:cluster{i32, dbl, "Data":dbl[]})  [unwired: 1 in]
      n53 = Bundle(0, w47, "Data"=w104) -> (w97:cluster{i32, dbl, "Data":dbl[]})  [unwired: 1 in]
      n54 = Bundle(0, w47, "Data"=w102) -> (w95:cluster{i32, dbl, "Data":dbl[]})  [unwired: 1 in]
      n55 = Bundle(0, w47, "Data"=w98) -> (w94:cluster{i32, dbl, "Data":dbl[]})  [unwired: 1 in]
      n56 = Bundle(0, w47, "Data"=w99) -> (w93:cluster{i32, dbl, "Data":dbl[]})  [unwired: 1 in]
      n57 = Bundle(0, w47, "Data"=w103) -> (w96:cluster{i32, dbl, "Data":dbl[]})  [unwired: 1 in]
      n58 = Bundle(0, w47, "Data"=w105) -> (w92:cluster{i32, dbl, "Data":dbl[]})  [unwired: 1 in]
      n59 = call-poly <vilib>:"Analog to Digital.vi"("data format (offset binary)"=w90, "full-scale range (pk-pk)"=256.0, "resolution (16 bit)"=8, "analog waveform"=w74) -> ("digital waveform"=w86:digitalwaveform)  [unwired: 4 in, 3 out]
      n60 = Or(x="stop", y="Run") -> (x .or. y?=w56:bool)
      n61 = local write "Capture Complete"(TRUE ("Capture Complete")) -> ()
      n62 = Build Array(w118, w117, w97, w96, w95, w94, w93, w92) -> (→"Analog Channels":cluster{i32, dbl, "Data":dbl[]}[])
      n63 = Bundle By Name("t0"=timestamp(0 s since 1904-01-01), "dt"=w47, "Y"=w86) -> (→"Port 0":digitalwaveform)  [unwired: 1 in]
      n64 = Wait (ms)(milliseconds to wait=u32 100) -> ()  [unwired: 1 out]
    }
    n65 = feedback-in #1(w26) -> ()
    "Capture Complete" <- FALSE ("Capture Complete")
  }
  n66 = call "PicoScope6000aClose.vi"("error in (no error)"=w5, "handle in"=w6) -> ()  [unwired: 8 in, 2 out]
